vi "LJM get and check exp config.vi"(0 "Working Directory In":path, 1 "App Name":string) -> (4 "Write To File":bool, 6 "Data File Prefix":string="data", 7 "Interval (ms)":u32=500, 8 "Scan Rate (Hz)":dbl=500.0 format="%.3f", 10 "Graph History":i32=1000 min=0, 11 "New Exp Config?":bool, 13 "Device Config File Name":string, 14 "Device Config Path":path, 15 "# Channels":i32=4, 16 "Disable Scaling":bool, 17 "Max File Size (Bytes)":i32=1048576, 18 "Channel Setup":T1={"+Ch"=["0", "1", "2", "3", "4", "5", "6", "7"], "-Ch"=["199", "199", "199", "199", "199", "199", "199", "199"], "Ranges"=[0, 0, 0, 0, 0, 0, 0, 0], "Scaling Equation"=["y=v0", "y=v1", "y=v2", "y=v3", "y=v4", "y=v5", "y=v6", "y=v7"], "Graph?"=[]} {"Ranges" items=["LJ_rgBIP10V", "LJ_rgBIP5V", "LJ_rgUNI5V", "LJ_rgUNI2P5V", "LJ_rgUNI1P25V", "LJ_rgBIP1V", "LJ_rgUNIP625V", "LJ_rgBIPP1V", "LJ_rgBIPP01V"]}, 19 "error out":errorcluster)   [LabVIEW 2025]
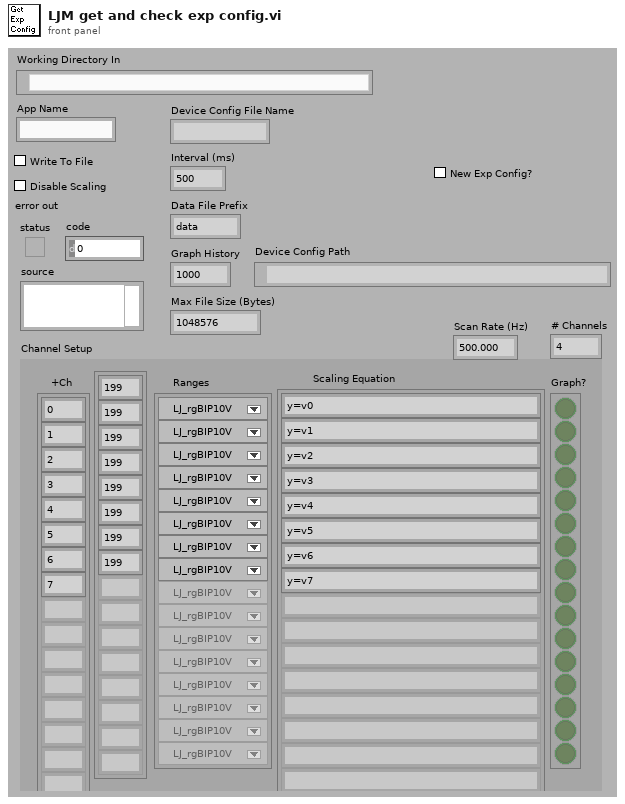
[diagram p1: front panel]
types:
  T1 = cluster{"+Ch":string[], "-Ch":string[], "Ranges":u16[], "Scaling Equation":string[], "Graph?":bool[]}
  T2 = enum16{"Left Button", "Center Button", "Right Button", "Window Close"}
  T3 = enum32{"existing file", "new file", "new or existing file", "existing dir", "new dir", "new or existing dir", "existing file (use LLBs)", "new file (use LLBs)", "new or existing file (use LLBs)", "new or existing file or directory (use LLBs)"}
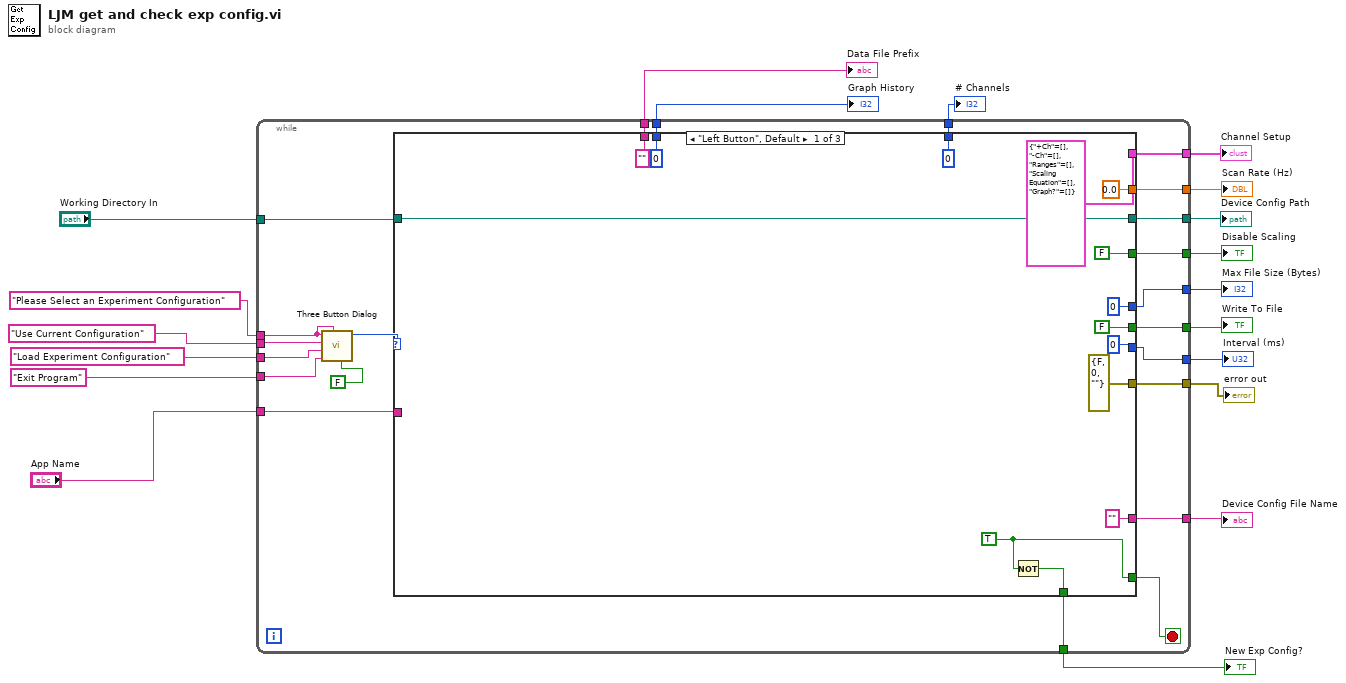
[diagram p0: block diagram]
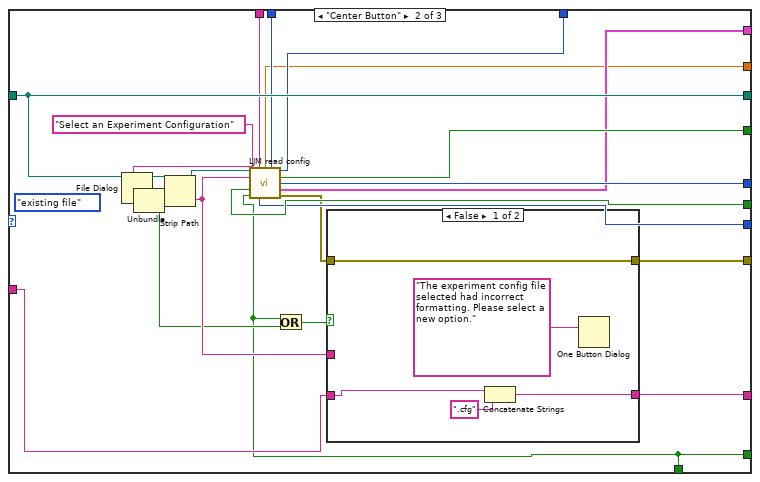
[diagram p2: hidden frame]
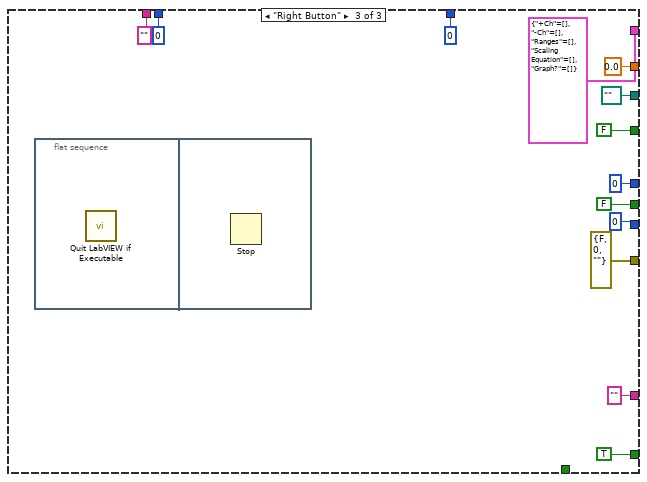
[diagram p4: hidden frame]
diagram:
  n1 = while {
    tunnel: "Working Directory In" -> [w41]
    tunnel: "App Name" -> [w40]
    tunnel: [w39] -> w17
    tunnel: "Use Current Configuration" ("F button name (\"Cancel\")") -> [w25]
    tunnel: "Load Experiment Configuration" ("T button name (\"OK\")") -> [w38]
    tunnel: "Please Select an Experiment Configuration" ("message") -> [w23]
    tunnel: [w36] -> w13
    tunnel: [w35] -> w12
    tunnel: [w34] -> w11
    tunnel: [w33] -> w10
    tunnel: [w32] -> w9
    tunnel: [w31] -> w8
    tunnel: [w30] -> w7
    tunnel: [w29] -> w6
    tunnel: [w28] -> w5
    tunnel: [w27] -> w4
    tunnel: [w26] -> w3
    tunnel: "Exit Program" ("Right Button Text (\"Cancel\")") -> [w24]
    tunnel: [w20] -> w1
    stop <- w21 stop-if-true
    n2 = call <vilib>:"Three Button Dialog.vi"("Allow user to close window? (TRUE)"=FALSE, "Window Title (\"\")"=w23, "Right Button Text (\"Cancel\")"=w24, "Center Button Text (\"No\")"=w38, "Left Button Text (\"Yes\")"=w25, "message"=w23) -> ("Which Button?"=w37:T2)  [unwired: 5 in]
    n3 = case shown="\"Left Button\", Default" w37 {
      tunnel: w41 -> [w42 w76 _]
      tunnel: w40 -> [_ w64 _]
      tunnel: [w42 w76 path "" ("Working Directory In")] -> w39
      tunnel: [FALSE ("Write To File") w74 FALSE ("Write To File")] -> w36
      tunnel: [u32 0 ("Interval (ms)") w73 u32 0 ("Interval (ms)")] -> w35
      tunnel: ["" ("Data File Prefix") w72 "" ("Data File Prefix")] -> w34
      tunnel: [0 ("Graph History") w71 0 ("Graph History")] -> w33
      tunnel: [0 ("# Channels") w70 0 ("# Channels")] -> w32
      tunnel: [FALSE ("Disable Scaling") w69 FALSE ("Disable Scaling")] -> w31
      tunnel: [0 ("Max File Size (Bytes)") w68 0 ("Max File Size (Bytes)")] -> w30
      tunnel: [T1 {"+Ch"=[], "-Ch"=[], "Ranges"=[], "Scaling Equation"=[], "Graph?"=[]} ("Channel Setup") w67 T1 {"+Ch"=[], "-Ch"=[], "Ranges"=[], "Scaling Equation"=[], "Graph?"=[]} ("Channel Setup")] -> w29
      tunnel: ["" ("name") w63 "" ("name")] -> w28
      tunnel: [errorcluster {"status"=FALSE, "code"=0, "source"=""} ("error out") w62 errorcluster {"status"=FALSE, "code"=0, "source"=""} ("error out")] -> w27
      tunnel: [0.0 ("Scan Rate (Hz)") w60 0.0 ("Scan Rate (Hz)")] -> w26
      tunnel: [w44 w57 TRUE ("Good Experiment Config")] -> w21
      tunnel: [w43 w57 _] -> w20
      frame "Left Button", Default {
        w44 = TRUE ("Good Experiment Config")
        n4 = Not(x=w44) -> (.not. x?=w43:bool)
      }
      frame "Center Button" {
        (unwired) T3."existing file" ("select mode (2)")
        n5 = File Dialog(7:"Select an Experiment Configuration" ("Substring"), 11:w76) -> (0:w56:errorcluster, 1:w58:bool, 3:w75:path)  [unwired: 5 in, 1 out]
        n6 = Unbundle(w56) -> ()  [unwired: 3 out]
        n7 = Strip Path(path=w75) -> (stripped path=w61:path, name=w65:string)
        n8 = call "LJM read config.vi"("Working Directory"=w61, "filename"=w65) -> ("Data File Prefix"=w72:string, "Scan Rate (Hz)"=w60:dbl, "Graph History"=w71:i32, "# Channels"=w70:i32, "Disable Scaling"=w69:bool, "Max File Size (Bytes)"=w68:i32, "Write To File"=w74:bool, "Channel Setup"=w67:T1, "Good Experiment Config"=w57:bool, "Interval (ms)"=w73:u32, "error out"=w66:errorcluster)  [unwired: 1 in, 2 out]
        n9 = Or(x=w57, y=w58) -> (x .or. y?=w59:bool)
        n10 = case shown="False" w59 {
          tunnel: w64 -> [w80 _]
          tunnel: [w79 w84] -> w63
          tunnel: w65 -> [_ w84]
          tunnel: w66 -> [w78 w83]
          tunnel: [w78 w83] -> w62
          frame False {
            n11 = Concatenate Strings(w80, ".cfg" ("string")) -> (w79:string)
            n12 = One Button Dialog(message="The experiment config file selected had incorrect formatting. Please select a new option.") -> ()  [unwired: 1 in, 1 out]
          }
          frame True {
          }
        }
      }
      frame "Right Button" {
        n13 = flat-sequence {
          frame #0 {
            n14 = call "Quit LabVIEW if Executable.vi"() -> ()  [unwired: 1 in]
          }
          frame #1 {
            n15 = Stop() -> ()  [unwired: 1 in]
          }
        }
      }
    }
  }
  "Device Config Path" <- w17
  "Device Config File Name" <- w5
  "error out" <- w4
  "Interval (ms)" <- w12
  "Write To File" <- w13
  "Data File Prefix" <- w11
  "Graph History" <- w10
  "# Channels" <- w9
  "Disable Scaling" <- w8
  "Max File Size (Bytes)" <- w7
  "Channel Setup" <- w6
  "Scan Rate (Hz)" <- w3
  "New Exp Config?" <- w1
